vi "CleanUp.vi"(8 "error in (no error)":errorcluster, 11 "object in":refnum<class "Base.lvclass">) -> (0 "error out":errorcluster, 3 "object out":refnum<class "Base.lvclass">)   [LabVIEW 2012, in "Base.lvclass"]
uses:
  Base.lvclass
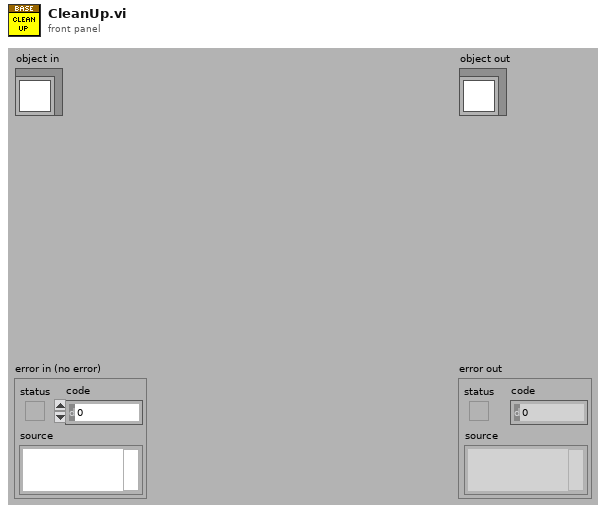
[diagram p1: front panel]
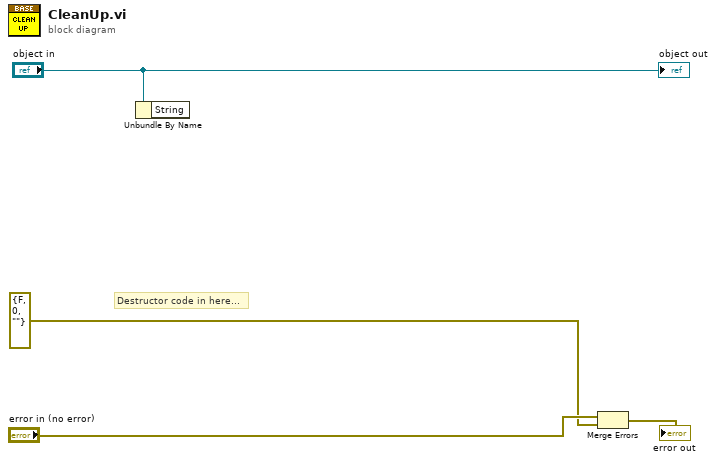
[diagram p0: block diagram]
diagram:
  # "Destructor code in here..."
  n1 = Unbundle By Name("object in") -> ()  [unwired: 1 out]
  n2 = Merge Errors("error in (no error)", errorcluster {"status"=FALSE, "code"=0, "source"=""} ("error in (no error)")) -> (→"error out":errorcluster)
  "object out" <- "object in"
